vi "exposureTimeErrorMessage.vi"(11 "errorIn":errorcluster) -> (2 "exposureTimeStatus":bool caption="Status")   [LabVIEW 2021]
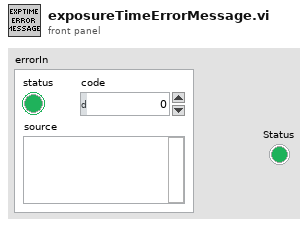
[diagram p1: front panel]
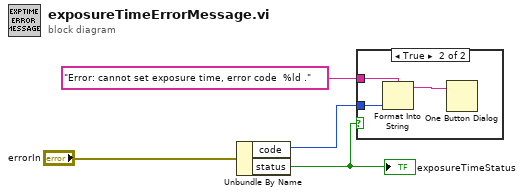
[diagram p0: block diagram]
diagram:
  n1 = Unbundle By Name("errorIn") -> ("code"=w4:i32, "status"=w1:bool)
  "exposureTimeStatus" <- w1
  n2 = case shown="True" w1 {
    tunnel: w4 -> [_ w7]
    tunnel: "Error: cannot set exposure time, error code  %ld ." ("format string") -> [_ w5]
    frame False {
    }
    frame True {
      n3 = Format Into String(format string=w5, w7) -> (resulting string=w6:string)  [unwired: 2 in, 1 out]
      n4 = One Button Dialog(message=w6) -> ()  [unwired: 1 in, 1 out]
    }
  }
